vi "Search_1D_Array(I32).vi"(0 "Array":i32[](array[numeric]), 2 "Element Data":i32, 3 "Start Index (0)":i32) -> (7 "Indicies of Elements":i32[](array[numeric]), 9 "Elements":i32[](array[numeric]))   [LabVIEW 2011]
doc: "Searches for all element data matches in array"
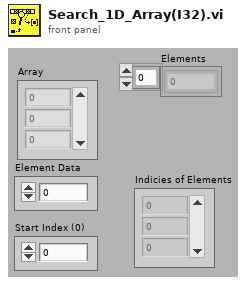
[diagram p1: front panel]
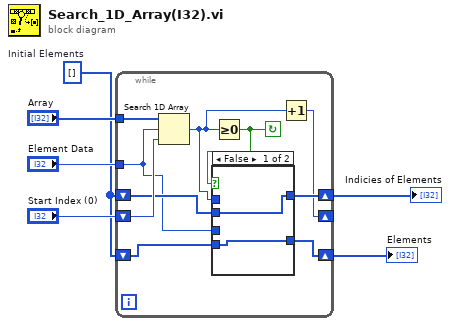
[diagram p0: block diagram]
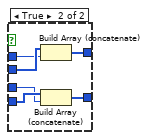
[diagram p2: hidden frame]
diagram:
  w1 = i32[] []  # Initial Elements
  n1 = while {
    shift-right: [w12] -> _
    shift-left: "Start Index (0)" -> [w16]
    shift-right: [w13] -> w3
    shift-left: w1 -> [w14]
    tunnel: "Array" -> [w15]
    tunnel: "Element Data" -> [w7]
    shift-right: [w10] -> w2
    shift-left: w1 -> [w11]
    stop <- w9 continue-if-true
    n2 = Search 1D Array(1D array=w15, element=w7, start index (0)=w16) -> (index of element=w8:i32)
    n3 = Greater Or Equal To 0?(x=w8) -> (x >= 0?=w9:bool)
    n4 = case shown="False" w9 {
      tunnel: w14 -> [w18 w24]
      tunnel: [w18 w23] -> w13
      tunnel: w11 -> [w17 w21]
      tunnel: [w17 w22] -> w10
      tunnel: w8 -> [_ w20]
      tunnel: w7 -> [_ w19]
      frame False {
      }
      frame True {
        n5 = Build Array (concatenate)(w24, w20) -> (w23:i32[])
        n6 = Build Array (concatenate)(w21, w19) -> (w22:i32[])
      }
    }
    n7 = Increment(x=w8) -> (x+1=w12:i32)
  }
  "Indicies of Elements" <- w3
  "Elements" <- w2
